vi "Panel Loop.vi"(8 "error in":errorcluster, 10 "panel":refnum<vi>, 11 "Material-Scheme in":refnum<class "Material-Scheme.lvclass">) -> (0 "error out":errorcluster, 3 "Material-Scheme out":refnum<class "Material-Scheme.lvclass">)   [LabVIEW 2021, in "TSC Material Theme.lvlib" / "Material-Scheme.lvclass"]
doc: "Apply coloring to all panes on the given Panel based on its item-tag data.\n\nTag Name: panel-level\nDefault: Surface\n\n<b>Code Developed By:</b>\nDaniel Coons\nTechnology Service Corporation\nwww.tsc.com/atcs"
uses:
  Material-Scheme.lvclass
  Material-Scheme.lvclass/Material-Scheme.ctl
  data member access/get surface.vi
  data member access/get background.vi
  data member access/get surfaceDim.vi
  data member access/get surfaceBright.vi
  data member access/get surfaceVariant.vi
  data member access/get surfaceContainerLowest.vi
  data member access/get surfaceContainerLow.vi
  data member access/get surfaceContainer.vi
  data member access/get surfaceContainerHigh.vi
  data member access/get surfaceContainerHighest.vi
  data member access/get inverseSurface.vi
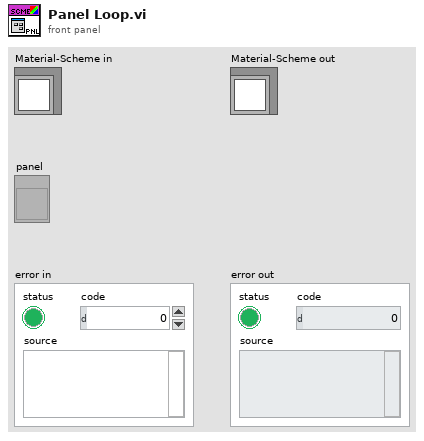
[diagram p1: front panel]
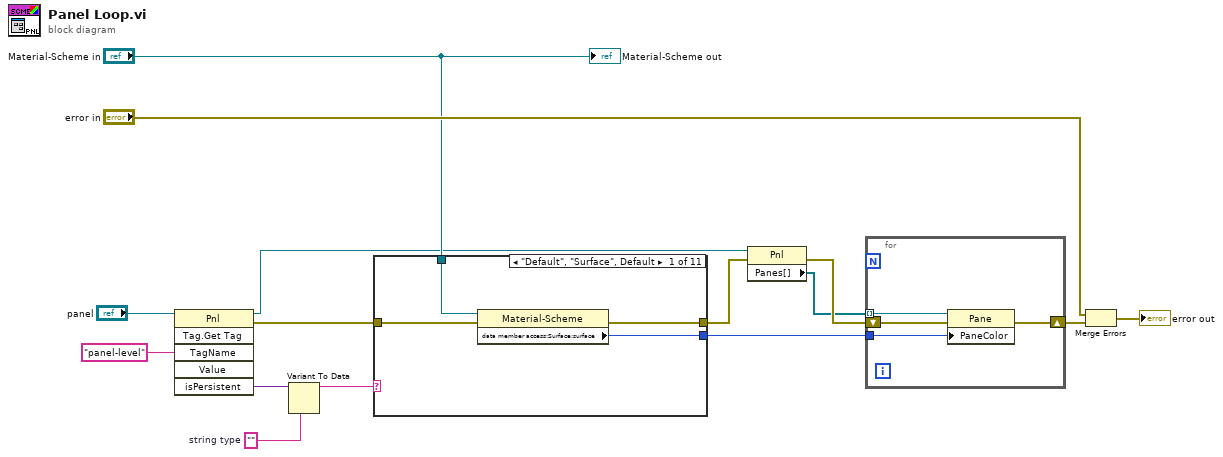
[diagram p0: block diagram]
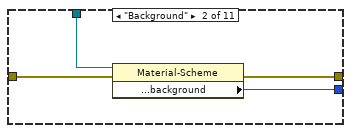
[diagram p2: hidden frame]
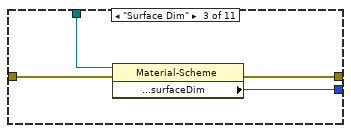
[diagram p3: hidden frame]
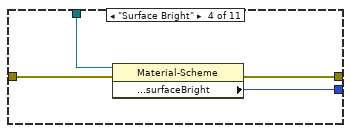
[diagram p4: hidden frame]
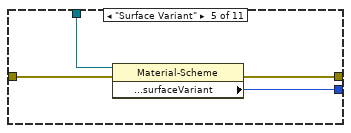
[diagram p5: hidden frame]
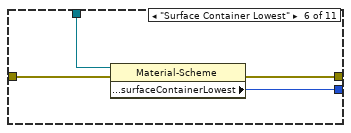
[diagram p6: hidden frame]
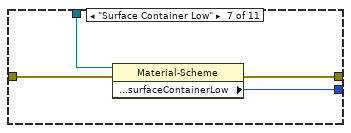
[diagram p7: hidden frame]
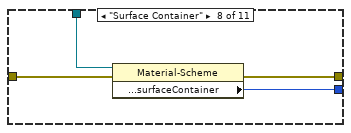
[diagram p8: hidden frame]
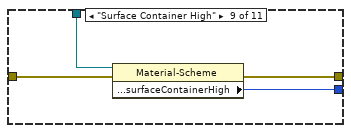
[diagram p9: hidden frame]
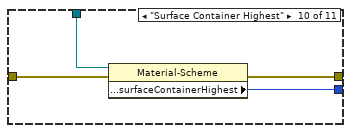
[diagram p10: hidden frame]
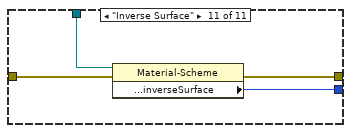
[diagram p11: hidden frame]
diagram:
  w6 = ""  # string type
  n1 = invoke class="Pnl" method="Tag.Get Tag"(reference="panel", "TagName"="panel-level" ("Tag Name")) -> (reference out=w2:refnum<vi>, error out=w12:errorcluster, "isPersistent"=w7:variant)  [unwired: 4 in, 3 out]
  n2 = Variant To Data(type=w6, Variant=w7) -> (data=w4:string)  [unwired: 1 in, 1 out]
  n3 = case shown="\"Default\", \"Surface\", Default" w4 {
    tunnel: "Material-Scheme in" -> [w17 w21 w25 w29 w33 w37 w41 w45 w49 w53 w57]
    tunnel: [w16 w20 w24 w28 w32 w36 w40 w44 w48 w52 w56] -> w3
    tunnel: w12 -> [w19 w23 w27 w31 w35 w39 w43 w47 w51 w55 w59]
    tunnel: [w18 w22 w26 w30 w34 w38 w42 w46 w50 w54 w58] -> w11
    frame "Default", "Surface", Default {
      n4 = property class="Material-Scheme"(reference=w17, error in=w19) -> (error out=w18:errorcluster, "data member access:Surface:surface"=w16:u32)  [unwired: 1 out]
    }
    frame "Background" {
      n5 = property class="Material-Scheme"(reference=w21, error in=w23) -> (error out=w22:errorcluster, "data member access:Surface:background"=w20:u32)  [unwired: 1 out]
    }
    frame "Surface Dim" {
      n6 = property class="Material-Scheme"(reference=w25, error in=w27) -> (error out=w26:errorcluster, "data member access:Surface:surfaceDim"=w24:u32)  [unwired: 1 out]
    }
    frame "Surface Bright" {
      n7 = property class="Material-Scheme"(reference=w29, error in=w31) -> (error out=w30:errorcluster, "data member access:Surface:surfaceBright"=w28:u32)  [unwired: 1 out]
    }
    frame "Surface Variant" {
      n8 = property class="Material-Scheme"(reference=w33, error in=w35) -> (error out=w34:errorcluster, "data member access:Surface:surfaceVariant"=w32:u32)  [unwired: 1 out]
    }
    frame "Surface Container Lowest" {
      n9 = property class="Material-Scheme"(reference=w37, error in=w39) -> (error out=w38:errorcluster, "data member access:Surface:surfaceContainerLowest"=w36:u32)  [unwired: 1 out]
    }
    frame "Surface Container Low" {
      n10 = property class="Material-Scheme"(reference=w41, error in=w43) -> (error out=w42:errorcluster, "data member access:Surface:surfaceContainerLow"=w40:u32)  [unwired: 1 out]
    }
    frame "Surface Container" {
      n11 = property class="Material-Scheme"(reference=w45, error in=w47) -> (error out=w46:errorcluster, "data member access:Surface:surfaceContainer"=w44:u32)  [unwired: 1 out]
    }
    frame "Surface Container High" {
      n12 = property class="Material-Scheme"(reference=w49, error in=w51) -> (error out=w50:errorcluster, "data member access:Surface:surfaceContainerHigh"=w48:u32)  [unwired: 1 out]
    }
    frame "Surface Container Highest" {
      n13 = property class="Material-Scheme"(reference=w53, error in=w55) -> (error out=w54:errorcluster, "data member access:Surface:surfaceContainerHighest"=w52:u32)  [unwired: 1 out]
    }
    frame "Inverse Surface" {
      n14 = property class="Material-Scheme"(reference=w57, error in=w59) -> (error out=w58:errorcluster, "data member access:Surface:inverseSurface"=w56:u32)  [unwired: 1 out]
    }
  }
  n15 = property class="Pnl"(reference=w2, error in=w11) -> (error out=w10:errorcluster, "Panes[]"=w1:refnum<vi>[])  [unwired: 1 out]
  n16 = for {
    tunnel: w3 -> [w61]
    tunnel: w1 -> [w60] mode=indexing
    shift-right: [w63] -> w13
    shift-left: w10 -> [w62]
    n17 = property class="Pane"(reference=w60, error in=w62, "PaneColor"=w61) -> (error out=w63:errorcluster)  [unwired: 1 out]
  }
  n18 = Merge Errors("error in", w13) -> (→"error out":errorcluster)
  "Material-Scheme out" <- "Material-Scheme in"
